vi "MerweScSigPts_GetWc_Single.vi"(9 "Element":i32, 11 "MerweScaledSigmaPts":T1) -> (3 "Wc_Value":dbl)   [LabVIEW 2019, in "Trajectory_Library.lvlib"]
doc: "Returns an element of the weight for each sigma point for the covariance.\n \nInputs:\n - MerweScaledSigmaPts -- data cluster\n - element -- Element of vector to return.\n\nOutputs:\n - Wc_Value -- The element I's weight for the covariance."
uses:
  Trajectory_Library.lvlib
  MERWE_SCALED_SIGMA_PTS.ctl
  <vilib>/Analysis/Matrix/Datatypes/RealMatrix.ctl
  <vilib>/Analysis/Matrix/NI_Matrix.lvlib
panel:
  # "<?, 1>"
  # "<?, 1>"
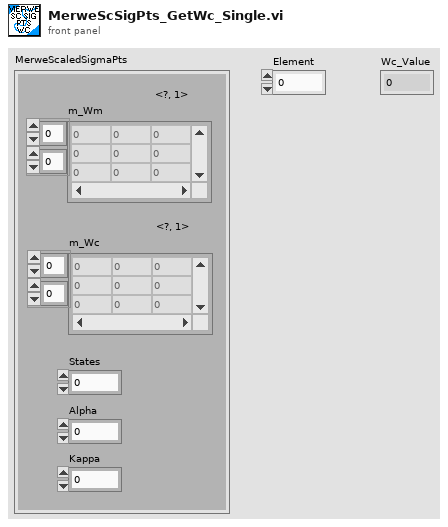
[diagram p1: front panel]
types:
  T1 = typedef "Trajectory_Library.lvlib/MERWE_SCALED_SIGMA_PTS.ctl" = cluster{"m_Wm":T2, "States":i32, "Alpha":dbl, "m_Wc":T2, "Kappa":i32}
  T2 = typedef "NI_Matrix.lvlib/RealMatrix.ctl" = dbl[][]
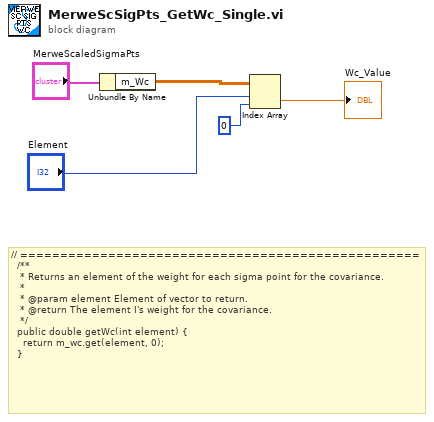
[diagram p0: block diagram]
diagram:
  # "// ==================================================\n  /**\n   * Returns an element of the weight for each sigma point for the covariance.\n   *\n   * @param element Element of vector to return.\n   * @return The element I's weight for the covariance.\n   */\n  public double getWc(int element) {\n    return m_wc.get(element, 0);\n  }"
  n1 = Unbundle By Name("MerweScaledSigmaPts") -> ("m_Wc"=w4:T2)
  n2 = Index Array(array=w4, index (row)="Element", index (col)=0) -> (element=→"Wc_Value":dbl)
